vi "ReadWaveformFile.vi"() -> ()   [LabVIEW 2015]
uses:
  <vilib>/Waveform/WDTFileIO.llb/Read Waveform from File.vi
panel:
  out "Waveform Graph":waveform(dbl)(graph)={"t0"=timestamp(0 s since 1904-01-01), "dt"=2.0, "Y"=array[1000 elements]}
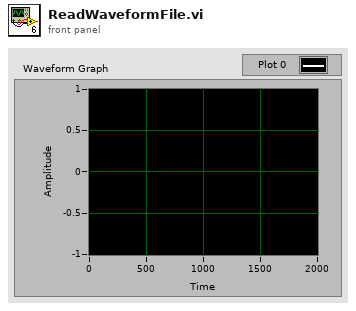
[diagram p1: front panel]
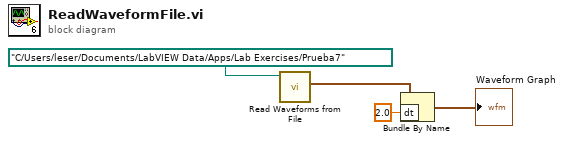
[diagram p0: block diagram]
diagram:
  n1 = call-poly <vilib>:"Read Waveforms from File.vi"("file path (dialog if empty)"=path "C:/Users/leser/Documents/LabVIEW Data/Apps/Lab Exercises/Prueba7") -> ("first waveform in record"=w4:waveform(dbl))  [unwired: 5 in, 3 out]
  n2 = Bundle By Name(cluster=w4, "dt"=2.0) -> (→"Waveform Graph":waveform(dbl))
